vi "PID.vi"() -> ()   [LabVIEW 2021]
uses:
  <vilib>/Instr/_visa.llb/VISA Configure Serial Port (Instr).vi
  <vilib>/ptbypt/NI_PtbyPt.lvlib
panel:
  out "error":i32
  out "ERROR":dbl(slide) scale=-5.0..5.0
  in  "PUERTO COM \nEN ARDUINO":refnum<visa-resource-name>
  out "PIN 3 PWM":i32
  in  "STEP":dbl(slide) scale=0.0..100.0
  out "Waveform Chart":dynamicdata(graph)
  out "A0":i32
  in  "kp":dbl=0.45
  in  "Ti":dbl=0.4
  in  "Td":dbl=0.2
  in  "T":dbl=0.012
  in  "OFF":bool
  # "ELECTROM@RK"
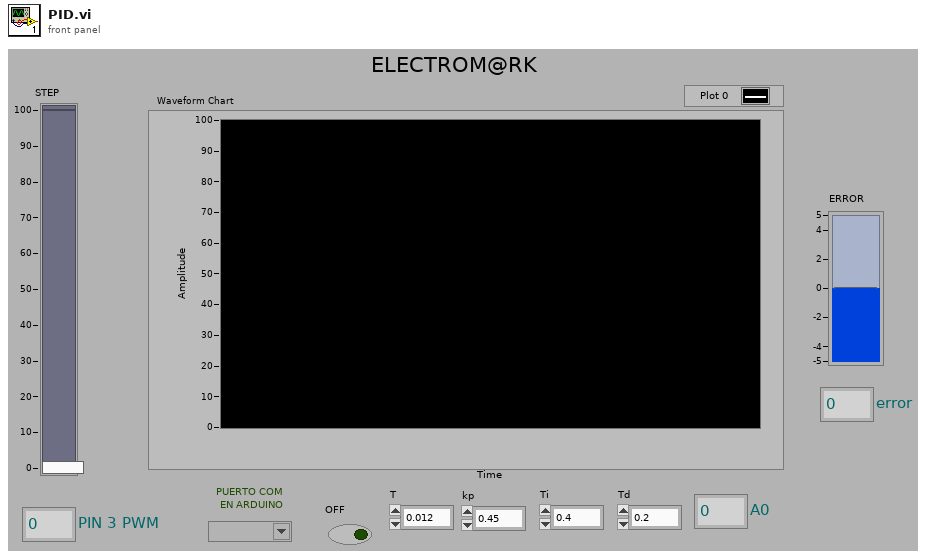
[diagram p1: front panel]
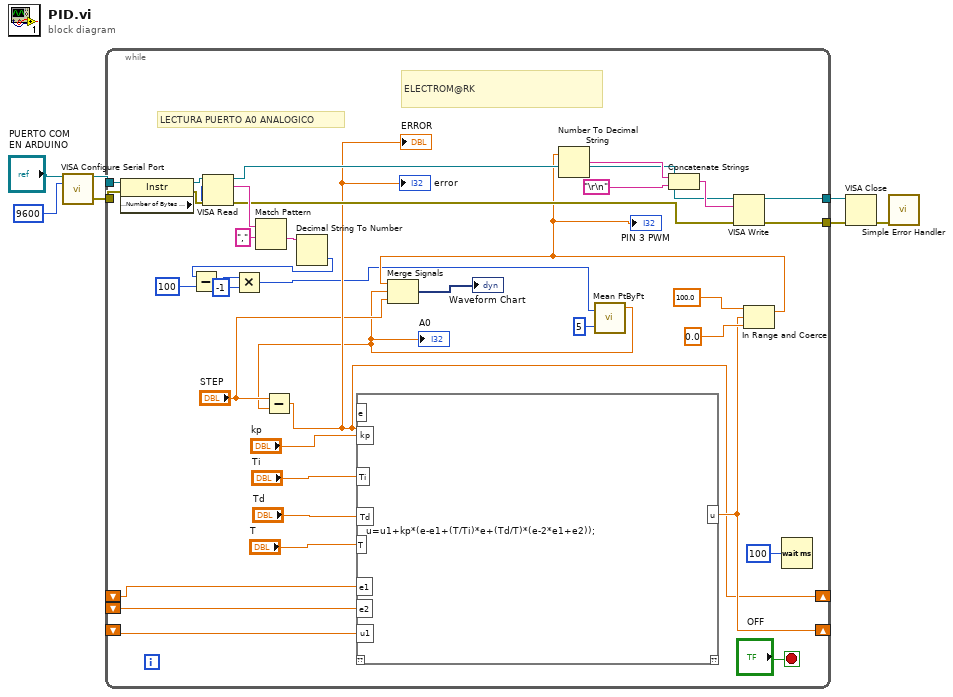
[diagram p0: block diagram]
diagram:
  n1 = call-poly "VISA Configure Serial Port"("VISA resource name"="PUERTO COM \nEN ARDUINO", "baud rate (9600)"=u32 9600) -> ("VISA resource name out"=w5:refnum<visa-resource-name>, "error out"=w4:errorcluster)  [unwired: 12 in]
  n2 = while {
    shift-right: [w18] -> _
    shift-left: _ -> [w45]
    shift-right: [w16] -> _
    shift-left: _ -> [w44]
    shift-left: _ -> [w43]
    tunnel: w5 -> [w22]
    tunnel: w4 -> [w21]
    tunnel: [w20] -> w2
    tunnel: [w19] -> w1
    stop <- "OFF" stop-if-true
    # "ELECTROM@RK"
    # "LECTURA PUERTO A0 ANALOGICO"
    n3 = property class="Instr"(reference=w22, error in=w21) -> (reference out=w34:refnum<visa-resource-name>, error out=w33:errorcluster, "Serial Settings:Number of Bytes at Serial Port"=w32:u32)
    n4 = VISA Read(VISA resource name=w34, byte count=w32, error in (no error)=w33) -> (VISA resource name out=w25:refnum<visa-resource-name>, read buffer=w31:string, error out=w24:errorcluster)  [unwired: 1 out]
    n5 = Match Pattern(string=w31, regular expression=",") -> (after substring=w29:string)  [unwired: 1 in, 3 out]
    n6 = Decimal String To Number(string=w29) -> (number=w11:i32)  [unwired: 2 in, 1 out]
    n7 = Subtract(x=w11, y=100) -> (x-y=w13:i32)
    n8 = Multiply(x=w13, y=-1) -> (x*y=w9:i32)
    n9 = call <vilib>:"Mean PtByPt.vi"("x"=w9, "sample length"=5) -> ("mean"=w8:dbl)  [unwired: 2 in, 1 out]
    "A0" <- w8
    n10 = Subtract(x="STEP", y=w8) -> (x-y=w16:dbl)
    "ERROR" <- w16
    "error" <- w16
    n11 = script code="u=u1+kp*(e-e1+(T/Ti)*e+(Td/T)*(e-2*e1+e2));"("kp"="kp", "Ti"="Ti", "Td"="Td", "T"="T", "e2"=w43, "e"=w16, "u1"=w45, "e1"=w44) -> ("u"=w18:dbl)  [unwired: 1 in, 1 out]
    n12 = In Range and Coerce(upper limit=100.0, x=w18, lower limit=0.0) -> (coerced(x)=w17:dbl)  [unwired: 1 out]
    "PIN 3 PWM" <- w17
    n13 = Merge Signals(w17, w8, "STEP") -> (→"Waveform Chart":dynamicdata)
    n14 = Number To Decimal String(number=w17) -> (decimal integer string=w27:string)  [unwired: 1 in]
    n15 = Concatenate Strings(w27, "\r\n") -> (w28:string)
    n16 = VISA Write(VISA resource name=w25, write buffer=w28, error in (no error)=w24) -> (VISA resource name out=w20:refnum<visa-resource-name>, error out=w19:errorcluster)  [unwired: 1 out]
    n17 = Wait (ms)(milliseconds to wait=u32 100) -> ()  [unwired: 1 out]
  }
  n18 = VISA Close(VISA resource name=w2, error in (no error)=w1) -> (error out=w3:errorcluster)
  n19 = call <vilib>:"Simple Error Handler.vi"("error in (no error)"=w3) -> ()  [unwired: 4 in, 5 out]
